vi "compareArrayData.vi"   [LabVIEW 2014]
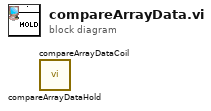
[diagram p0: block diagram]
diagram:
  n1 = call "compareArrayDataHold.vi"() -> ()  [unwired: 10 in, 2 out]
  n2 = call "compareArrayDataCoil.vi"() -> ()  [unwired: 10 in, 2 out]
